vi "03TRM800_GetScopeshot.vi"() -> ()   [LabVIEW 2015]
panel:
  out "Array":u16[](array[numeric])
  out "element":bool
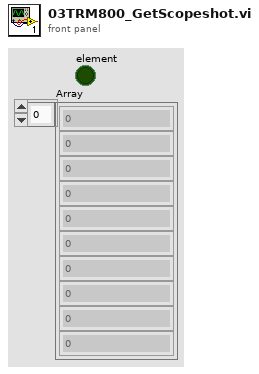
[diagram p1: front panel]
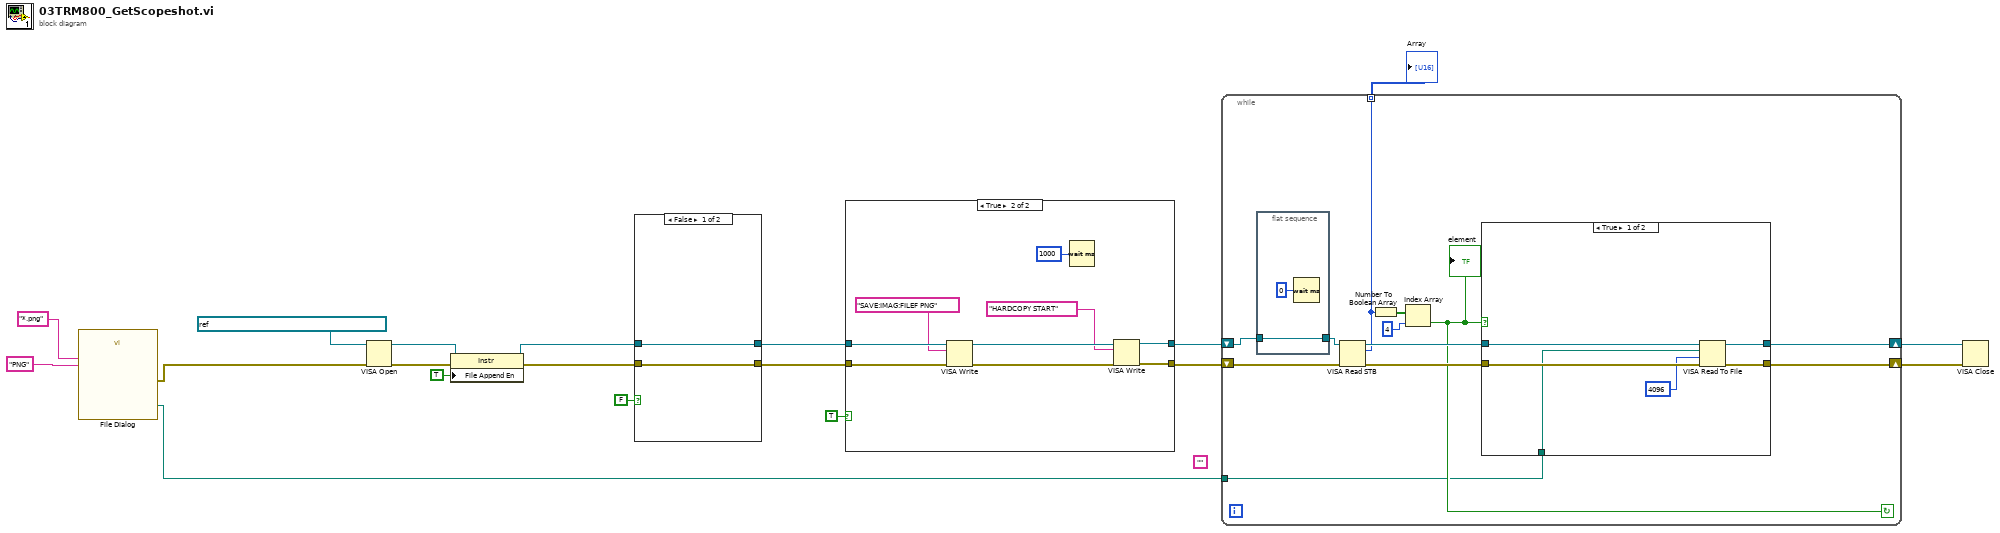
[diagram p0: block diagram]
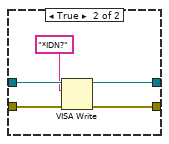
[diagram p4: hidden frame]
diagram:
  (unwired) ""
  n1 = call "File Dialog"("pattern (all files)"="*.png", "pattern label"="PNG") -> ("selected path"=w3:path, "error out"=w4:errorcluster)  [unwired: 10 in, 2 out]
  n2 = VISA Open(error in (no error)=w4, VISA resource name=refnum<visa-resource-name> "USB0::0x0699::0x03A3::C030456::INSTR") -> (VISA resource name=w8:refnum<visa-resource-name>, error out=w9:errorcluster)  [unwired: 3 in]
  n3 = property class="Instr"(reference=w8, error in=w9, "File Append En"=TRUE ("Message Based Settings:File Append Enable")) -> (reference out=w7:refnum<visa-resource-name>, error out=w6:errorcluster)
  n4 = case shown="False" FALSE {
    tunnel: [w21 w24] -> w15
    tunnel: w7 -> [w21 w26]
    tunnel: [w20 w23] -> w14
    tunnel: w6 -> [w20 w25]
    frame False {
    }
    frame True {
      n5 = VISA Write(VISA resource name=w26, write buffer="*IDN?", error in (no error)=w25) -> (VISA resource name out=w24:refnum<visa-resource-name>, error out=w23:errorcluster)  [unwired: 1 out]
    }
  }
  n6 = case shown="True" TRUE {
    tunnel: w15 -> [w28 w37]
    tunnel: w14 -> [w27 w36]
    tunnel: [w28 w31] -> w13
    tunnel: [w27 w32] -> w12
    frame False {
    }
    frame True {
      n7 = VISA Write(VISA resource name=w37, write buffer="SAVE:IMAG:FILEF PNG", error in (no error)=w36) -> (VISA resource name out=w34:refnum<visa-resource-name>, error out=w33:errorcluster)  [unwired: 1 out]
      n8 = Wait (ms)(milliseconds to wait=u32 1000) -> ()  [unwired: 1 out]
      n9 = VISA Write(VISA resource name=w34, write buffer="HARDCOPY START", error in (no error)=w33) -> (VISA resource name out=w31:refnum<visa-resource-name>, error out=w32:errorcluster)  [unwired: 1 out]
    }
  }
  n10 = while {
    shift-right: [w46] -> w17
    shift-left: w13 -> [w40]
    shift-right: [w45] -> w16
    shift-left: w12 -> [w49]
    tunnel: [w39] -> w10 mode=indexing
    tunnel: w3 -> [w38]
    stop <- w42 continue-if-true
    n11 = flat-sequence {
      tunnel: [w51] -> w41
      tunnel: w40 -> [w51]
      frame #0 {
        n12 = Wait (ms)(milliseconds to wait=u32 0) -> ()  [unwired: 1 out]
      }
    }
    n13 = VISA Read STB(8:w49, 11:w41) -> (0:w47:errorcluster, 2:w39:u16, 3:w48:refnum<visa-resource-name>)
    n14 = Number To Boolean Array(number=w39) -> (Boolean array=w44:bool[])
    n15 = Index Array(array=w44, index=4) -> (element=w42:bool)
    "element" <- w42
    n16 = case shown="True" w42 {
      tunnel: w48 -> [w57 w59]
      tunnel: w47 -> [w56 w58]
      tunnel: [w53 w59] -> w46
      tunnel: [w54 w58] -> w45
      tunnel: w38 -> [w52 _]
      frame True {
        n17 = VISA Read To File(8:w56, 9:u32 4096 ("byte count"), 10:w52, 11:w57) -> (0:w54:errorcluster, 3:w53:refnum<visa-resource-name>)  [unwired: 1 out]
      }
      frame False {
      }
    }
  }
  "Array" <- w10
  n18 = VISA Close(VISA resource name=w17, error in (no error)=w16) -> ()  [unwired: 1 out]
